vi "Simulate Triangle Signal.vi"(8 "error in (no error)":errorcluster) -> (0 "error out":errorcluster, 3 "Triangle with Uniform Noise":dynamicdata(graph))   [LabVIEW 2023, in "Scope Simulated CFGs.lvlib" / "Fetch Waveforms CFG.lvclass"]
uses:
  Fetch Waveforms CFG.lvclass
  Fetch Waveforms CFG.lvclass/Fetch Waveforms CFG.ctl
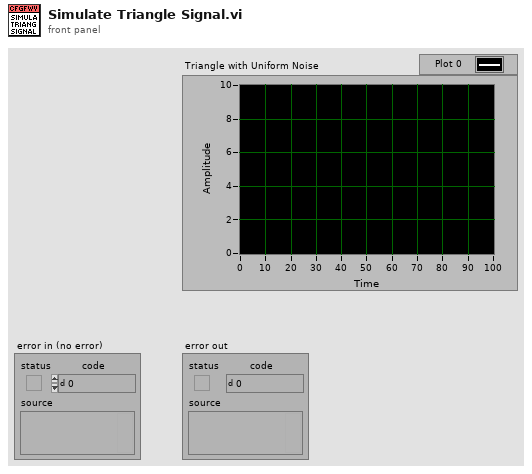
[diagram p1: front panel]
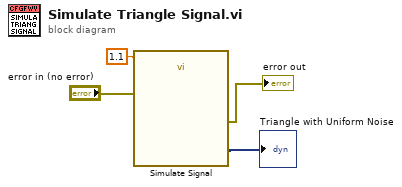
[diagram p0: block diagram]
diagram:
  n1 = call "Simulate Signal"("Offset"=1.1, "error in (no error)"="error in (no error)") -> ("Triangle with Uniform Noise"=→"Triangle with Uniform Noise":dynamicdata, "error out"=→"error out":errorcluster)  [unwired: 12 in]
